vi "Example System Functions.vi"   [LabVIEW 2014]
uses:
  <vilib>/regexp/Match Regular Expression.xnode
  <vilib>/Utility/file.llb/Write To Spreadsheet File (DBL).vi
  <vilib>/Utility/file.llb/Read From Spreadsheet File (DBL).vi
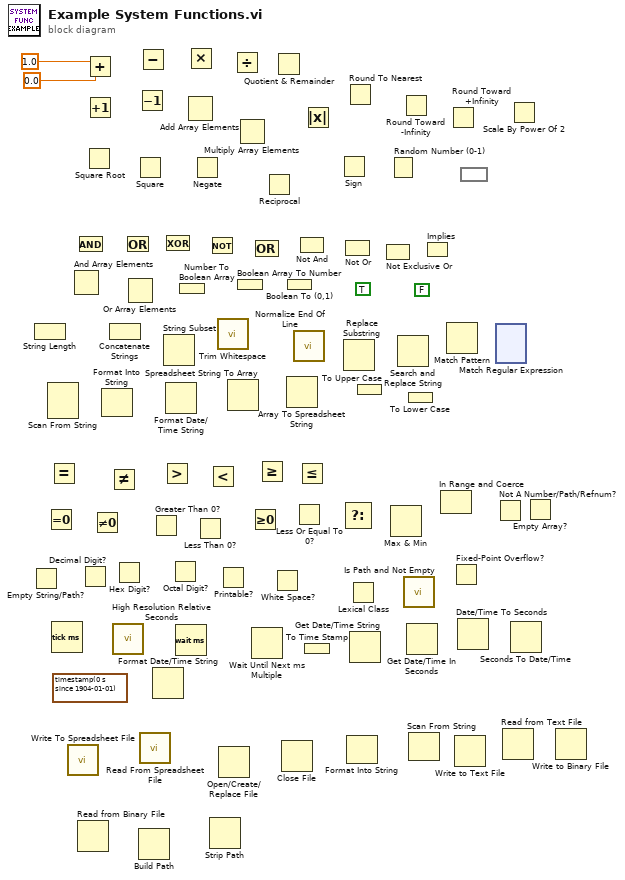
[diagram p0: block diagram]
diagram:
  (unwired) timestamp(0 s since 1904-01-01)
  (unwired) FALSE
  (unwired) TRUE
  n1 = Empty String/Path?() -> ()  [unwired: 1 in, 1 out]
  n2 = String Length() -> ()  [unwired: 1 in, 1 out]
  n3 = Equal To 0?() -> ()  [unwired: 1 in, 1 out]
  n4 = Scan From String() -> ()  [unwired: 6 in, 3 out]
  n5 = Equal?() -> ()  [unwired: 2 in, 1 out]
  n6 = Tick Count (ms)() -> ()  [unwired: 1 out]
  n7 = call-poly <vilib>:"Write To Spreadsheet File.vi"() -> ()  [unwired: 8 in, 1 out]
  n8 = And Array Elements() -> ()  [unwired: 1 in, 1 out]
  n9 = And() -> ()  [unwired: 2 in, 1 out]
  n10 = Read from Binary File() -> ()  [unwired: 6 in, 4 out]
  n11 = Decimal Digit?() -> ()  [unwired: 1 in, 1 out]
  n12 = Square Root() -> ()  [unwired: 1 in, 1 out]
  n13 = Add(x=1.0, y=0.0) -> ()  [unwired: 1 out]
  n14 = Increment() -> ()  [unwired: 1 in, 1 out]
  n15 = Not Equal To 0?() -> ()  [unwired: 1 in, 1 out]
  n16 = Format Into String() -> ()  [unwired: 4 in, 2 out]
  n17 = Not Equal?() -> ()  [unwired: 2 in, 1 out]
  n18 = Concatenate Strings() -> ()  [unwired: 2 in, 1 out]
  n19 = call <vilib>:"High Resolution Relative Seconds.vi"() -> ()  [unwired: 1 out]
  n20 = Hex Digit?() -> ()  [unwired: 1 in, 1 out]
  n21 = Or() -> ()  [unwired: 2 in, 1 out]
  n22 = Or Array Elements() -> ()  [unwired: 1 in, 1 out]
  n23 = Square() -> ()  [unwired: 1 in, 1 out]
  n24 = Decrement() -> ()  [unwired: 1 in, 1 out]
  n25 = Subtract() -> ()  [unwired: 2 in, 1 out]
  n26 = Build Path() -> ()  [unwired: 2 in, 1 out]
  n27 = call-poly <vilib>:"Read From Spreadsheet File.vi"() -> ()  [unwired: 7 in, 5 out]
  n28 = Greater Than 0?() -> ()  [unwired: 1 in, 1 out]
  n29 = Format Date/Time String() -> ()  [unwired: 3 in, 1 out]
  n30 = Greater?() -> ()  [unwired: 2 in, 1 out]
  n31 = Exclusive Or() -> ()  [unwired: 2 in, 1 out]
  n32 = String Subset() -> ()  [unwired: 3 in, 1 out]
  n33 = Format Date/Time String() -> ()  [unwired: 3 in, 1 out]
  n34 = Octal Digit?() -> ()  [unwired: 1 in, 1 out]
  n35 = Wait (ms)() -> ()  [unwired: 1 in, 1 out]
  n36 = Number To Boolean Array() -> ()  [unwired: 1 in, 1 out]
  n37 = Add Array Elements() -> ()  [unwired: 1 in, 1 out]
  n38 = Multiply() -> ()  [unwired: 2 in, 1 out]
  n39 = Negate() -> ()  [unwired: 1 in, 1 out]
  n40 = Less Than 0?() -> ()  [unwired: 1 in, 1 out]
  n41 = Not() -> ()  [unwired: 1 in, 1 out]
  n42 = Less?() -> ()  [unwired: 2 in, 1 out]
  n43 = Strip Path() -> ()  [unwired: 1 in, 2 out]
  n44 = call <vilib>:"Trim Whitespace.vi"() -> ()  [unwired: 2 in, 1 out]
  n45 = Printable?() -> ()  [unwired: 1 in, 1 out]
  n46 = Open/Create/Replace File() -> ()  [unwired: 6 in, 3 out]
  n47 = Spreadsheet String To Array() -> ()  [unwired: 4 in, 1 out]
  n48 = Divide() -> ()  [unwired: 2 in, 1 out]
  n49 = Boolean Array To Number() -> ()  [unwired: 1 in, 1 out]
  n50 = Multiply Array Elements() -> ()  [unwired: 1 in, 1 out]
  n51 = Greater Or Equal To 0?() -> ()  [unwired: 1 in, 1 out]
  n52 = Wait Until Next ms Multiple() -> ()  [unwired: 1 in, 1 out]
  n53 = Compound Arithmetic op=OR() -> ()  [unwired: 2 in, 1 out]
  n54 = Greater Or Equal?() -> ()  [unwired: 2 in, 1 out]
  n55 = Reciprocal() -> ()  [unwired: 1 in, 1 out]
  n56 = White Space?() -> ()  [unwired: 1 in, 1 out]
  n57 = Quotient & Remainder() -> ()  [unwired: 2 in, 2 out]
  n58 = Close File() -> ()  [unwired: 2 in, 2 out]
  n59 = Boolean To (0,1)() -> ()  [unwired: 1 in, 1 out]
  n60 = Array To Spreadsheet String() -> ()  [unwired: 3 in, 1 out]
  n61 = call <vilib>:"Normalize End Of Line.vi"() -> ()  [unwired: 8 in, 1 out]
  n62 = Less Or Equal To 0?() -> ()  [unwired: 1 in, 1 out]
  n63 = Not And() -> ()  [unwired: 2 in, 1 out]
  n64 = Less Or Equal?() -> ()  [unwired: 2 in, 1 out]
  n65 = To Time Stamp() -> ()  [unwired: 1 in, 1 out]
  n66 = Absolute Value() -> ()  [unwired: 1 in, 1 out]
  n67 = Sign() -> ()  [unwired: 1 in, 1 out]
  n68 = Not Or() -> ()  [unwired: 2 in, 1 out]
  n69 = Select() -> ()  [unwired: 3 in, 1 out]
  n70 = Replace Substring() -> ()  [unwired: 4 in, 2 out]
  n71 = Round To Nearest() -> ()  [unwired: 1 in, 1 out]
  n72 = Format Into String ("Format Into File")() -> ()  [unwired: 4 in, 2 out]
  n73 = Lexical Class() -> ()  [unwired: 1 in, 1 out]
  n74 = Get Date/Time String() -> ()  [unwired: 3 in, 2 out]
  n75 = To Upper Case() -> ()  [unwired: 1 in, 1 out]
  n76 = Not Exclusive Or() -> ()  [unwired: 2 in, 1 out]
  n77 = Random Number (0-1)() -> ()  [unwired: 1 out]
  n78 = Max & Min() -> ()  [unwired: 2 in, 2 out]
  n79 = Search and Replace String() -> ()  [unwired: 8 in, 4 out]
  n80 = Round Toward -Infinity() -> ()  [unwired: 1 in, 1 out]
  n81 = call <vilib>:"Is Path and Not Empty.vi"() -> ()  [unwired: 5 in, 1 out]
  n82 = To Lower Case() -> ()  [unwired: 1 in, 1 out]
  n83 = Get Date/Time In Seconds() -> ()  [unwired: 1 out]
  n84 = Scan From String ("Scan From File")() -> ()  [unwired: 5 in, 2 out]
  n85 = Implies() -> ()  [unwired: 2 in, 1 out]
  n86 = In Range and Coerce() -> ()  [unwired: 3 in, 2 out]
  n87 = Match Pattern() -> ()  [unwired: 3 in, 4 out]
  n88 = Round Toward +Infinity() -> ()  [unwired: 1 in, 1 out]
  n89 = Fixed-Point Overflow?() -> ()  [unwired: 1 in, 1 out]
  n90 = Write to Text File() -> ()  [unwired: 4 in, 3 out]
  n91 = Date/Time To Seconds() -> ()  [unwired: 2 in, 1 out]
  n92 = expression code=""() -> ()  [unwired: 1 in, 1 out]
  n93 = Not A Number/Path/Refnum?() -> ()  [unwired: 1 in, 1 out]
  n94 = xnode ("Match Regular Expression")() -> ()  [unwired: 6 in, 5 out]
  n95 = Read from Text File() -> ()  [unwired: 4 in, 4 out]
  n96 = Scale By Power Of 2() -> ()  [unwired: 2 in, 1 out]
  n97 = Seconds To Date/Time() -> ()  [unwired: 2 in, 1 out]
  n98 = Empty Array?() -> ()  [unwired: 1 in, 1 out]
  n99 = Write to Binary File() -> ()  [unwired: 6 in, 3 out]
